vi "Configure Thermocouple.vi"(0 "VISA resource name":refnum<visa-resource-name>="GPIB0::16::INSTR", 1 "Thermocouple Type (1: K)":u16(ring)=1 items=["J", "K", "T", "E", "R", "S", "B", "N"], 2 "Reference Junction Type (0: Simulated)":u16(ring) items=["Simulated", "Internal", "External"], 3 "Simulated Reference Temperature (23 deg C)":dbl=23.0, 4 "Enable Open Detector? (False)":bool, 5 "error in (no error)":errorcluster, 6 "Scan List (Empty)":string) -> (14 "VISA resource name out":refnum<visa-resource-name>, 19 "error out":errorcluster)   [LabVIEW 2020, in "Keithley 27XX.lvlib"]
doc: "This VI sets the temperature transducer to Thermocouple. Additionally, it configures attributes related to thermocouple based temperature measurements.\n\nNote: \n(1) Configure Measurement.vi must be called <B>before</B> running this VI.\n\n(2) This VI will only work if the DMM is in Temperature Measurement mode."
uses:
  Keithley 27XX.lvlib
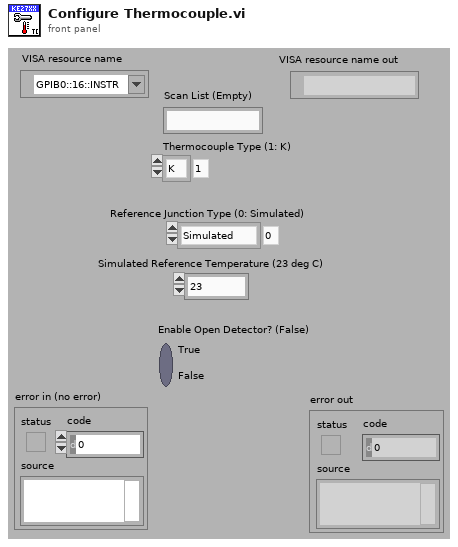
[diagram p1: front panel]
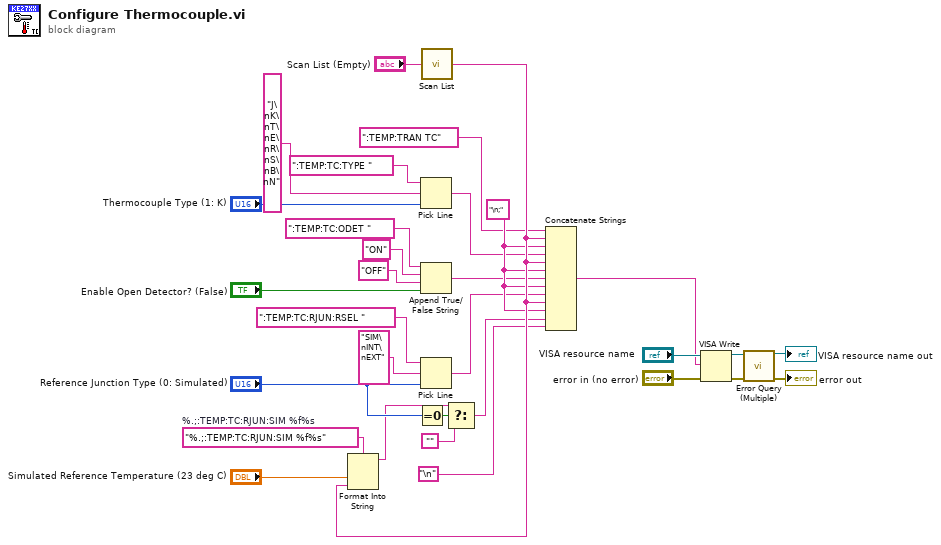
[diagram p0: block diagram]
diagram:
  w11 = "\n;" ("string")
  w16 = "%.;:TEMP:TC:RJUN:SIM %f%s"  # %.;:TEMP:TC:RJUN:SIM %f%s
  n1 = Equal To 0?(x="Reference Junction Type (0: Simulated)") -> (x = 0?=w5:bool)
  n2 = Pick Line(string ("")=":TEMP:TC:TYPE ", multi-line string="J\nK\nT\nE\nR\nS\nB\nN", line index="Thermocouple Type (1: K)") -> (output string=w9:string)
  n3 = Append True/False String(1:"Enable Open Detector? (False)", 2:"OFF" ("false string"), 3:"ON" ("true string"), 4:":TEMP:TC:ODET ") -> (0:w8:string)
  n4 = Pick Line(string ("")=":TEMP:TC:RJUN:RSEL ", multi-line string="SIM\nINT\nEXT", line index="Reference Junction Type (0: Simulated)") -> (output string=w7:string)
  n5 = call "Scan List.vi"("Scan List (Empty)"="Scan List (Empty)") -> ("Scan List Out"=w31:string)  [unwired: 14 in]
  n6 = Format Into String(format string=w16, "Simulated Reference Temperature (23 deg C)", w31) -> (resulting string=w3:string)  [unwired: 2 in, 1 out]
  n7 = Select(t=w3, s=w5, f="") -> (s? t:f=w2:string)
  n8 = Concatenate Strings(":TEMP:TRAN TC", w31, w11, w9, w31, w11, w8, w11, w7, w31, w11, w2, "\n") -> (w19:string)
  n9 = VISA Write(VISA resource name="VISA resource name", write buffer=w19, error in (no error)="error in (no error)") -> (VISA resource name out=w15:refnum<visa-resource-name>, error out=w14:errorcluster)  [unwired: 1 out]
  n10 = call "Error Query (Multiple).vi"("VISA resource name"=w15, "error in (no error)"=w14) -> ("VISA resource name out"=→"VISA resource name out":refnum<visa-resource-name>, "error out"=→"error out":errorcluster)  [unwired: 10 in, 2 out]
